vi "GlobalVar.vi"() -> ()   [LabVIEW 2010]
panel:
  in  "stop execution":bool
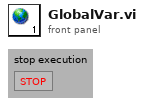
[diagram p1: front panel]
diagram:
